vi "Counter U16 With Init.vi"(6 "reset":bool, 9 "increment":bool, 10 "inintial value":u16) -> (2 "count":u16)   [LabVIEW 2020]
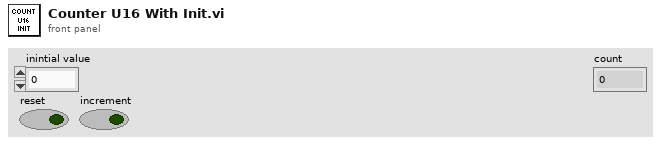
[diagram p1: front panel]
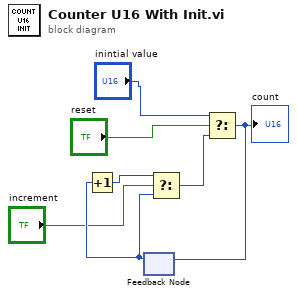
[diagram p0: block diagram]
diagram:
  n1 = feedback #1() -> (w2:u16)  [unwired: 1 in]
  n2 = Increment(x=w2) -> (x+1=w3:u16)
  n3 = Select(t=w3, s="increment", f=w2) -> (s? t:f=w5:u16)
  n4 = Select(t="inintial value", s="reset", f=w5) -> (s? t:f=w4:u16)
  "count" <- w4
  n5 = feedback-in #1(w4) -> ()
